vi "Read Port.vi"(0 "Arduino in":refnum<class "Arduino.lvclass">, 5 "VISA resource name":refnum<visa-resource-name>, 7 "Port":dbl, 11 "error in (no error)":errorcluster) -> (4 "Arduino out":refnum<class "Arduino.lvclass">, 6 "VISA resource name 2":refnum<visa-resource-name>, 8 "Binary Number":T1, 10 "Response":string, 15 "error out":errorcluster)   [LabVIEW 2020, in "Arduino.lvclass"]
uses:
  Arduino.lvclass
  a4ea8719-085e-44e5-bbf3-3b2cfe874b76.vi
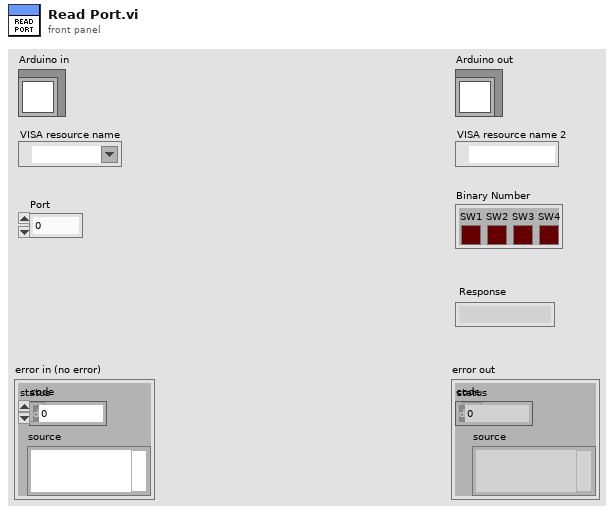
[diagram p1: front panel]
types:
  T1 = cluster{"SW1":bool, "SW2":bool, "SW3":bool, "SW4":bool, "[4]":bool, "[5]":bool, "[6]":bool, "[7]":bool, "[8]":bool}
  T2 = enum16{"Write", "Read", "Config", "Reset", "Close"}
  T3 = cluster{"[0]":bool, "[1]":bool, "[2]":bool, "[3]":bool, "[4]":bool, "[5]":bool, "[6]":bool, "[7]":bool, "[8]":bool}
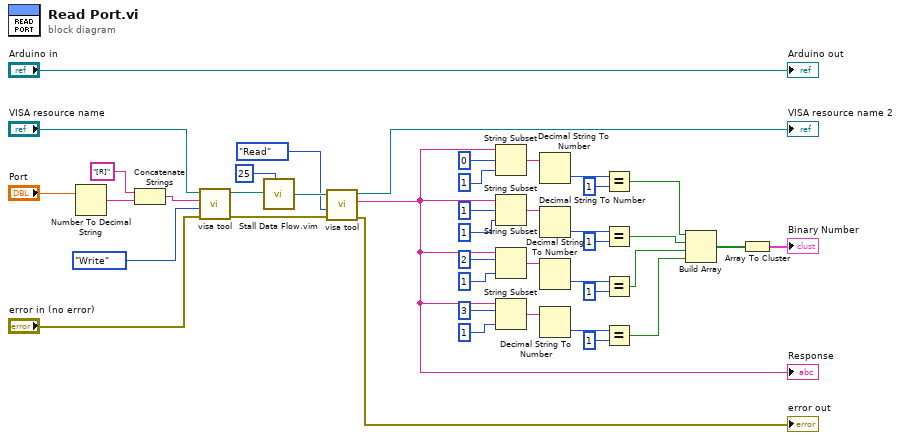
[diagram p0: block diagram]
diagram:
  n1 = Number To Decimal String(number="Port") -> (decimal integer string=w3:string)  [unwired: 1 in]
  n2 = Concatenate Strings("[R]" ("string"), w3) -> (w2:string)
  n3 = call "visa tool.vi"("error in (no error)"="error in (no error)", "Opciones"=T2."Write", "Write"=w2, "VISA com port"="VISA resource name") -> ("error out"=w33:errorcluster, "VISA com port 2"=w37:refnum<visa-resource-name>)  [unwired: 5 in, 1 out]
  n4 = call "Stall Data Flow.vim"("value in"=w37, "milliseconds to wait"=u32 25) -> ("value out"=w36:refnum<visa-resource-name>)  [unwired: 1 out]
  n5 = call "visa tool.vi"("error in (no error)"=w33, "Opciones"=T2."Read", "VISA com port"=w36) -> ("error out"=→"error out":errorcluster, "Read"=w30:string, "VISA com port 2"=→"VISA resource name 2":refnum<visa-resource-name>)  [unwired: 6 in]
  "Response" <- w30
  n6 = String Subset(string=w30, offset (0)=0, length (rest)=1 ("length (rest)")) -> (substring=w21:string)
  n7 = String Subset(string=w30, offset (0)=1, length (rest)=1 ("length (rest)")) -> (substring=w20:string)
  n8 = String Subset(string=w30, offset (0)=2, length (rest)=1 ("length (rest)")) -> (substring=w19:string)
  n9 = String Subset(string=w30, offset (0)=3, length (rest)=1 ("length (rest)")) -> (substring=w18:string)
  n10 = Decimal String To Number(string=w21) -> (number=w17:i32)  [unwired: 2 in, 1 out]
  n11 = Decimal String To Number(string=w20) -> (number=w12:i32)  [unwired: 2 in, 1 out]
  n12 = Decimal String To Number(string=w19) -> (number=w11:i32)  [unwired: 2 in, 1 out]
  n13 = Decimal String To Number(string=w18) -> (number=w10:i32)  [unwired: 2 in, 1 out]
  n14 = Equal?(x=w17, y=1) -> (x = y?=w9:bool)
  n15 = Equal?(x=w12, y=1) -> (x = y?=w8:bool)
  n16 = Equal?(x=w11, y=1) -> (x = y?=w7:bool)
  n17 = Equal?(x=w10, y=1) -> (x = y?=w6:bool)
  n18 = Build Array(w9, w8, w7, w6) -> (w5:bool[])
  n19 = Array To Cluster(array=w5) -> (cluster=→"Binary Number":T3)
  "Arduino out" <- "Arduino in"
